vi "pixel_to_mm.vi"() -> (0 "mm/pixel":dbl)   [LabVIEW 2020]
panel:
  out "Pixel distance":dbl format="%#_8g"
  in  "distance in mm":dbl=0.2
  in  "P2":dbl[](array[numeric])=[1231.0, 300.0]
  in  "P1":dbl[](array[numeric])=[761.0, 274.0]
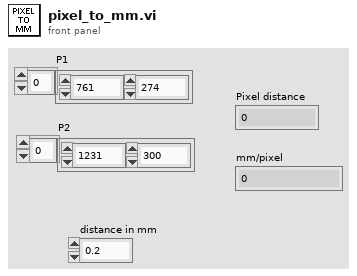
[diagram p1: front panel]
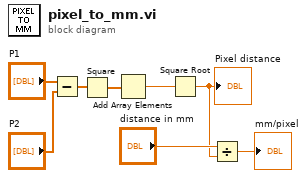
[diagram p0: block diagram]
diagram:
  n1 = Subtract(x="P1", y="P2") -> (x-y=w6:dbl[])
  n2 = Square(x=w6) -> (x^2=w5:dbl[])
  n3 = Add Array Elements(numeric array=w5) -> (sum=w4:dbl)
  n4 = Square Root(x=w4) -> (sqrt(x)=w1:dbl)
  "Pixel distance" <- w1
  n5 = Divide(x="distance in mm", y=w1) -> (x/y=→"mm/pixel":dbl)
